vi "OpenPrompt.vi"(9 "Container State":T1, 11 "Prompt VI Ref":refnum<vi>) -> ()   [LabVIEW 2019, in "ExpandVertical.xctl"]
uses:
  ExpandVertical.xctl
  <vilib>/_xctls/Container State.ctl
  <vilib>/_xctls/XControlSupport.lvlib
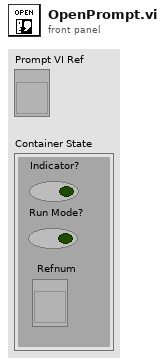
[diagram p1: front panel]
types:
  T1 = typedef "XControlSupport.lvlib/Container State.ctl" = cluster{"Indicator?":bool, "Run Mode?":bool, " Refnum":refnum<vi>}
  T2 = enum32{"Invalid", "Standard", "Closed", "Hidden", "Minimized", "Maximized"}
  T3 = typedef "LVRectTypeDef.ctl" = cluster{"Left":i16, "Top":i16, "Right":i16, "Bottom":i16}
  T4 = cluster{"left":i16, "top":i16, "right":i16, "bottom":i16}
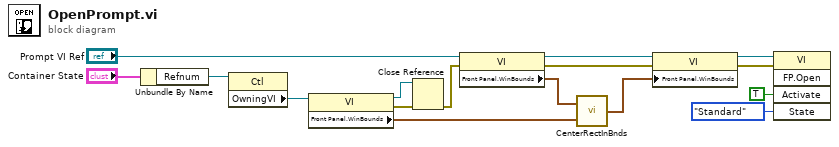
[diagram p0: block diagram]
diagram:
  n1 = Unbundle By Name("Container State") -> ("Refnum"=w6:refnum<vi>)
  n2 = property class="Ctl"(reference=w6) -> ("OwningVI"=w5:refnum<vi>)  [unwired: 1 in, 2 out]
  n3 = property class="VI"(reference=w5) -> (reference out=w2:refnum<vi>, error out=w3:errorcluster, "Front Panel.WinBounds"=w4:T3)  [unwired: 1 in]
  n4 = Close Reference(reference=w2, error in (no error)=w3) -> (error out=w1:errorcluster)
  n5 = property class="VI"(reference="Prompt VI Ref", error in=w1) -> (reference out=w16:refnum<vi>, error out=w15:errorcluster, "Front Panel.WinBounds"=w14:T3)
  n6 = call <vilib>:"CenterRectInBnds.vi"("bounds"=w4, "rect"=w14) -> ("centered rect"=w13:T4)
  n7 = property class="VI"(reference=w16, error in=w15, "Front Panel.WinBounds"=w13) -> (reference out=w10:refnum<vi>, error out=w9:errorcluster)
  n8 = invoke class="VI" method="FP.Open"(reference=w10, error in=w9, "Activate"=TRUE ("Activate?"), "State"=T2."Standard") -> ()  [unwired: 1 in, 5 out]
